vi "Pre Launch Init.vi"(11 "eActor in":refnum<class "eActor.lvclass">) -> (0 "error out":errorcluster, 3 "eActor out":refnum<class "eActor.lvclass">)   [LabVIEW 2015, in "AMS UI.lvlib" / "eActor.lvclass"]
doc: "(<B>Filename</B>: Actor Framework.lvlib:Actor.lvclass:Pre Launch Init.vi)\n\nDefines behavior that occurs after the Launch Actor method is invoked but before the actor's Actor Core method begins running.\n\nThe Pre Launch Init method is guaranteed to finish before the Launch Actor method returns to its caller and before the actor itself receives any messages. Any references that the Pre Launch Init method obtains are guaranteed to have the same lifetime as the actor itself. Any errors that the Pre Launch Init method returns will abort the launch.\n\nBy default, this method does nothing. A descendant class may override it to define behavior."
uses:
  eActor.lvclass
  <vilib>/ActorFramework/Actor/Actor.lvclass/Actor.ctl
  <vilib>/ActorFramework/Message Enqueuer/Message Enqueuer.lvclass/Message Enqueuer.ctl
  eActor.lvclass/eActor.ctl
  <vilib>/ActorFramework/Message Enqueuer/Init from Existing Queue.vi
  <vilib>/ActorFramework/Actor/Actor.lvclass
  <vilib>/ActorFramework/Message Enqueuer/Message Enqueuer.lvclass
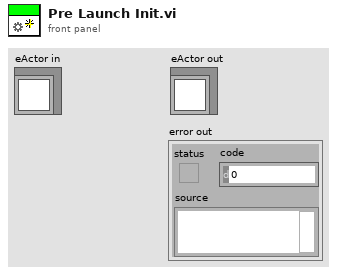
[diagram p1: front panel]
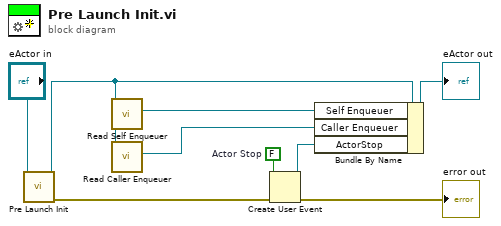
[diagram p0: block diagram]
diagram:
  w6 = FALSE  # Actor Stop
  n1 = call-parent "Pre Launch Init.vi"("Actor in"="eActor in") -> ("error out"=w7:errorcluster, "Actor out"=w3:refnum<class "eActor.lvclass">)  [unwired: 9 in]
  n2 = call <vilib>:"Read Self Enqueuer.vi"("Actor"=w3) -> ("Self Enqueuer"=w4:refnum<class "Message Enqueuer.lvclass">)  [unwired: 10 in]
  n3 = call <vilib>:"Read Caller Enqueuer.vi"("Actor"=w3) -> ("Caller Enqueuer"=w1:refnum<class "Message Enqueuer.lvclass">)  [unwired: 10 in]
  n4 = Create User Event(user event datatype=w6, error in=w7) -> (user event=w2:refnum<user-event>, error out=→"error out":errorcluster)
  n5 = Bundle By Name(cluster=w3, "Self Enqueuer"=w4, "Caller Enqueuer"=w1, "ActorStop"=w2) -> (→"eActor out":refnum<class "eActor.lvclass">)
